vi "Trauma Box Controller.vi"() -> ()   [LabVIEW 2020]
uses:
  epl-vi-lib/Utility VIs/Buttons/KCheckmarkBoolean.ctl
  epl-vi-lib/Utility VIs/Controls/KBackground Gradient/KBackground Gradient.xctl
  Typedefs/TB-Parameters.ctl
  Typedefs/TB-Slack State.ctl
  epl-vi-lib/PXI DAQ VIs/AIDI/Typedefs/AIDI-Action.ctl
  epl-vi-lib/PXI DAQ VIs/AODO/Typedefs/AODO-Action.ctl
  Typedefs/TB-State Enum.ctl
  <vilib>/Analysis/baseanly.llb/Mean (DBL).vi
  <vilib>/Analysis/5stat.llb/RMS (DBL).vi
  epl-vi-lib/Utility VIs/Math VIs/Linear to dB (scalar).vi
  <vilib>/Analysis/NI_AALPro.lvlib
  <vilib>/Analysis/NI_AALBase.lvlib
panel:
  out "Exposure":errorcluster
  out "Crown":errorcluster
  in  "Waveform":u16(ring)=2 items=["Noise", "File", "Tone"]
  in  "dB SPL":dbl=100.0
  in  "Duration (min)":dbl=120.0
  in  "Tab Control":enum32{"Tone", "Noise", "File"}(tab)
  in  "Frequency (kHz)":dbl=8.0
  in  "High cutoff (kHz)":dbl=16.0
  in  "Low cutoff (kHz)":dbl=8.0
  in  "refWAV":path caption="Ref"
  in  "WAVfile":path
  in  "Cal Log":path=path "C:/Data/Trauma Box/Trauma Box Calibration Log.txt"
  out "Pistonphone Factor":dbl=102.0 caption="Calibrator Voltage\n(dB rms re 1 uV)"
  in  "B&K Mic Gain":dbl=20.0
  in  "Display":enum32{"Page 1", "Page 2"}(tab)
  out "ma":dbl=99.37258874088361 caption="average" format="%.1f"
  out "Starts":i32
  out "Overload 2":bool caption="Overload"
  in  "Fine Control":dbl(slide) caption="Fine Adjust (dB)" scale=-6.0..6.0
  out "Spectrum":waveform(dbl)(graph)
  out "Waveform":waveform(dbl)(graph)
  out "dB SPL rms":dbl=99.37258874088361 format="%.2f"
  out "Gauge":dbl(knob)=99.37258874088361 scale=80.0..130.0
  out "Elapsed time":string
  out "SPL History":cluster{dbl[], dbl[]}[](graph)
  out "Expected":string="Expected value = 102"
  in  "micCorrFile":path
  in  "Use mic correction":T1 caption="Apply mic frequency correction (if you're unsure, then no)"
  out "Calibration Log":string[][](table)
  out "Overload":bool
  out "Calibrator Voltage\n(dB rms re 1 uV)":dbl=-inf
  out "Pistonphone\nWaveform":dbl[](graph)
  in  "Wizard":T2(tab)
  in  "START":bool
  in  "EXIT":bool
  in  "Use previous":bool
  in  "Remeasure":bool
  in  "Pistonphone measure":bool
  in  "Next":bool
  in  "To Crown adjust":bool
  in  "Start Crown":bool
  in  "Stop Crown":bool
  in  "Start Trauma":bool
  in  "Stop Trauma":bool
  in  "Finished":bool
  in  "User ID":string
  in  "Gradient":dbl(xcontrol)
  # "dB SPL"
  # "Press START to begin\nPress EXIT to quit"
  # "Step 1 Pistonphone correction"
  # "Step 1 Pistonphone correction\n    \n--Put ref mic into pistonphone\n--Make sure B&K gain is correct"
  # "Step 2 Put microphone in cage. It's going to get loud! Close the booth door before continuing."
  # "Step 3 Adjust amplifier until SPL is correct, then hit \"Stop\" button:"
  # "Step 4: Noise Exposure\n1. Put animal(s) in cage\n2. Set duration,\n3. Press START"
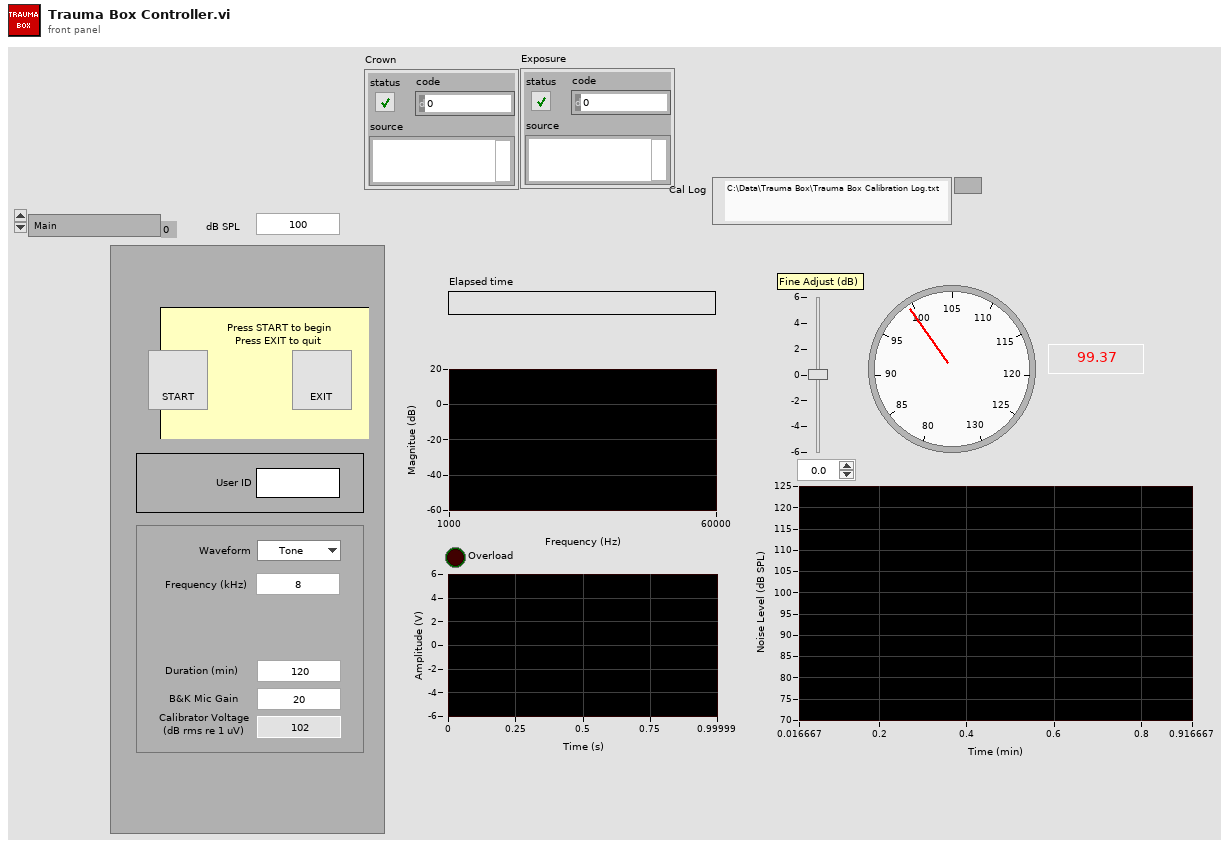
[diagram p1: front panel]
types:
  T1 = typedef "KCheckmarkBoolean.ctl" = bool
  T2 = enum32{"Main", "Pistonphone query", "Pistonphone measure", "Mic in cage", "Adjust Crown", "Animal in cage"}
  T3 = typedef "TB-Slack State.ctl" = cluster{"access_token":string, "bot id":string, "users":cluster{"id":string, "always":bool}[], "chan id":string}
  T4 = typedef "TB-Parameters.ctl" = cluster{"Low cutoff (kHz)":dbl, "High cutoff (kHz)":dbl, "Duration (min)":dbl, "dB SPL":dbl, "Waveform":enum16{"Noise", "File", "Tone"}, "WAVfile":path, "refWav":path, "use mic correction":bool, "micCorrFile":path, "Pistonphone Level (dB SPL)":dbl, "Sampling rate (Hz)":dbl, "Buffer length (s)":dbl, "Stream mic":bool, "Fine adjust":cluster{"Max":dbl, "Min":dbl}, "Mic gain":dbl, "atten":dbl, "resol (Hz)":dbl, "navgs":i32, "Allow Slack":bool, "max starts":i32, "Freq (kHz)":dbl, "Tma (s)":dbl, "Streamed":cluster{"Device":string, "Name":string}[], "Drive":string, "Speaker":string, "Mic":string}
  T5 = cluster{bool, "Exposure parameters":T4, "Slack":T3}
  T6 = typedef "AIDI-Action.ctl" = enum16{"Configure", "Initialize", "Start", "Read", "Clean up", "Init & Start", "Config & Test", "Position"}
  T7 = typedef "AODO-Action.ctl" = enum16{"Configure", "Initialize", "Start", "Write", "Clean up", "Init & Start", "Config & Test", "Position", "Set AO Gains", "Zero"}
  T8 = typedef "TB-Runtime state.ctl" = cluster{"stimfile":T9, "stream mic?":bool, "Fs":dbl, "ID":string, "micCorr":dbl[], "navg":i32, "r2sum":dbl[], "expose":bool, "spectra/frame":i32, "pts/spectra":i32, "nacq":i32, "init error":bool, "max starts":i32, "num starts":i32, "Setup":T10, "toneIndex":i32, "LastN":dbl[], "fine":dbl, "imic":i32, "stream":refnum<file>, "names":string[]}
  T9 = typedef "Sound File Refnum.ctl" = refnum<file>
  T10 = typedef "TB-Setup Log.ctl" = cluster{"Pistonphone factor":dbl, "Fine adjust":dbl, "Actual dB SPL":dbl, "Freq":dbl[], "Mag":dbl[]}
  T11 = typedef "TB-Stimulus State.ctl" = cluster{"filelen":i32, "stimfile":T9, "stimfile?":bool, "Fs":dbl, "Npts":i32, "stimfileend":bool, "atten":dbl, "AO":i32[]}
  T12 = typedef "TB-Log.ctl" = cluster{"Slack":T3, "entries":string[]}
  T13 = typedef "TB-Mic Queue.ctl" = refnum<queue>
  T14 = typedef "TB-State Enum.ctl" = enum16{"Main", "Pistonphone query", "Pistonphone measure", "Mic in cage", "Adjust Crown", "Animal in cage"}
  T15 = cluster{"notification":bool, "Parameters out":T4, "Slack":T3}
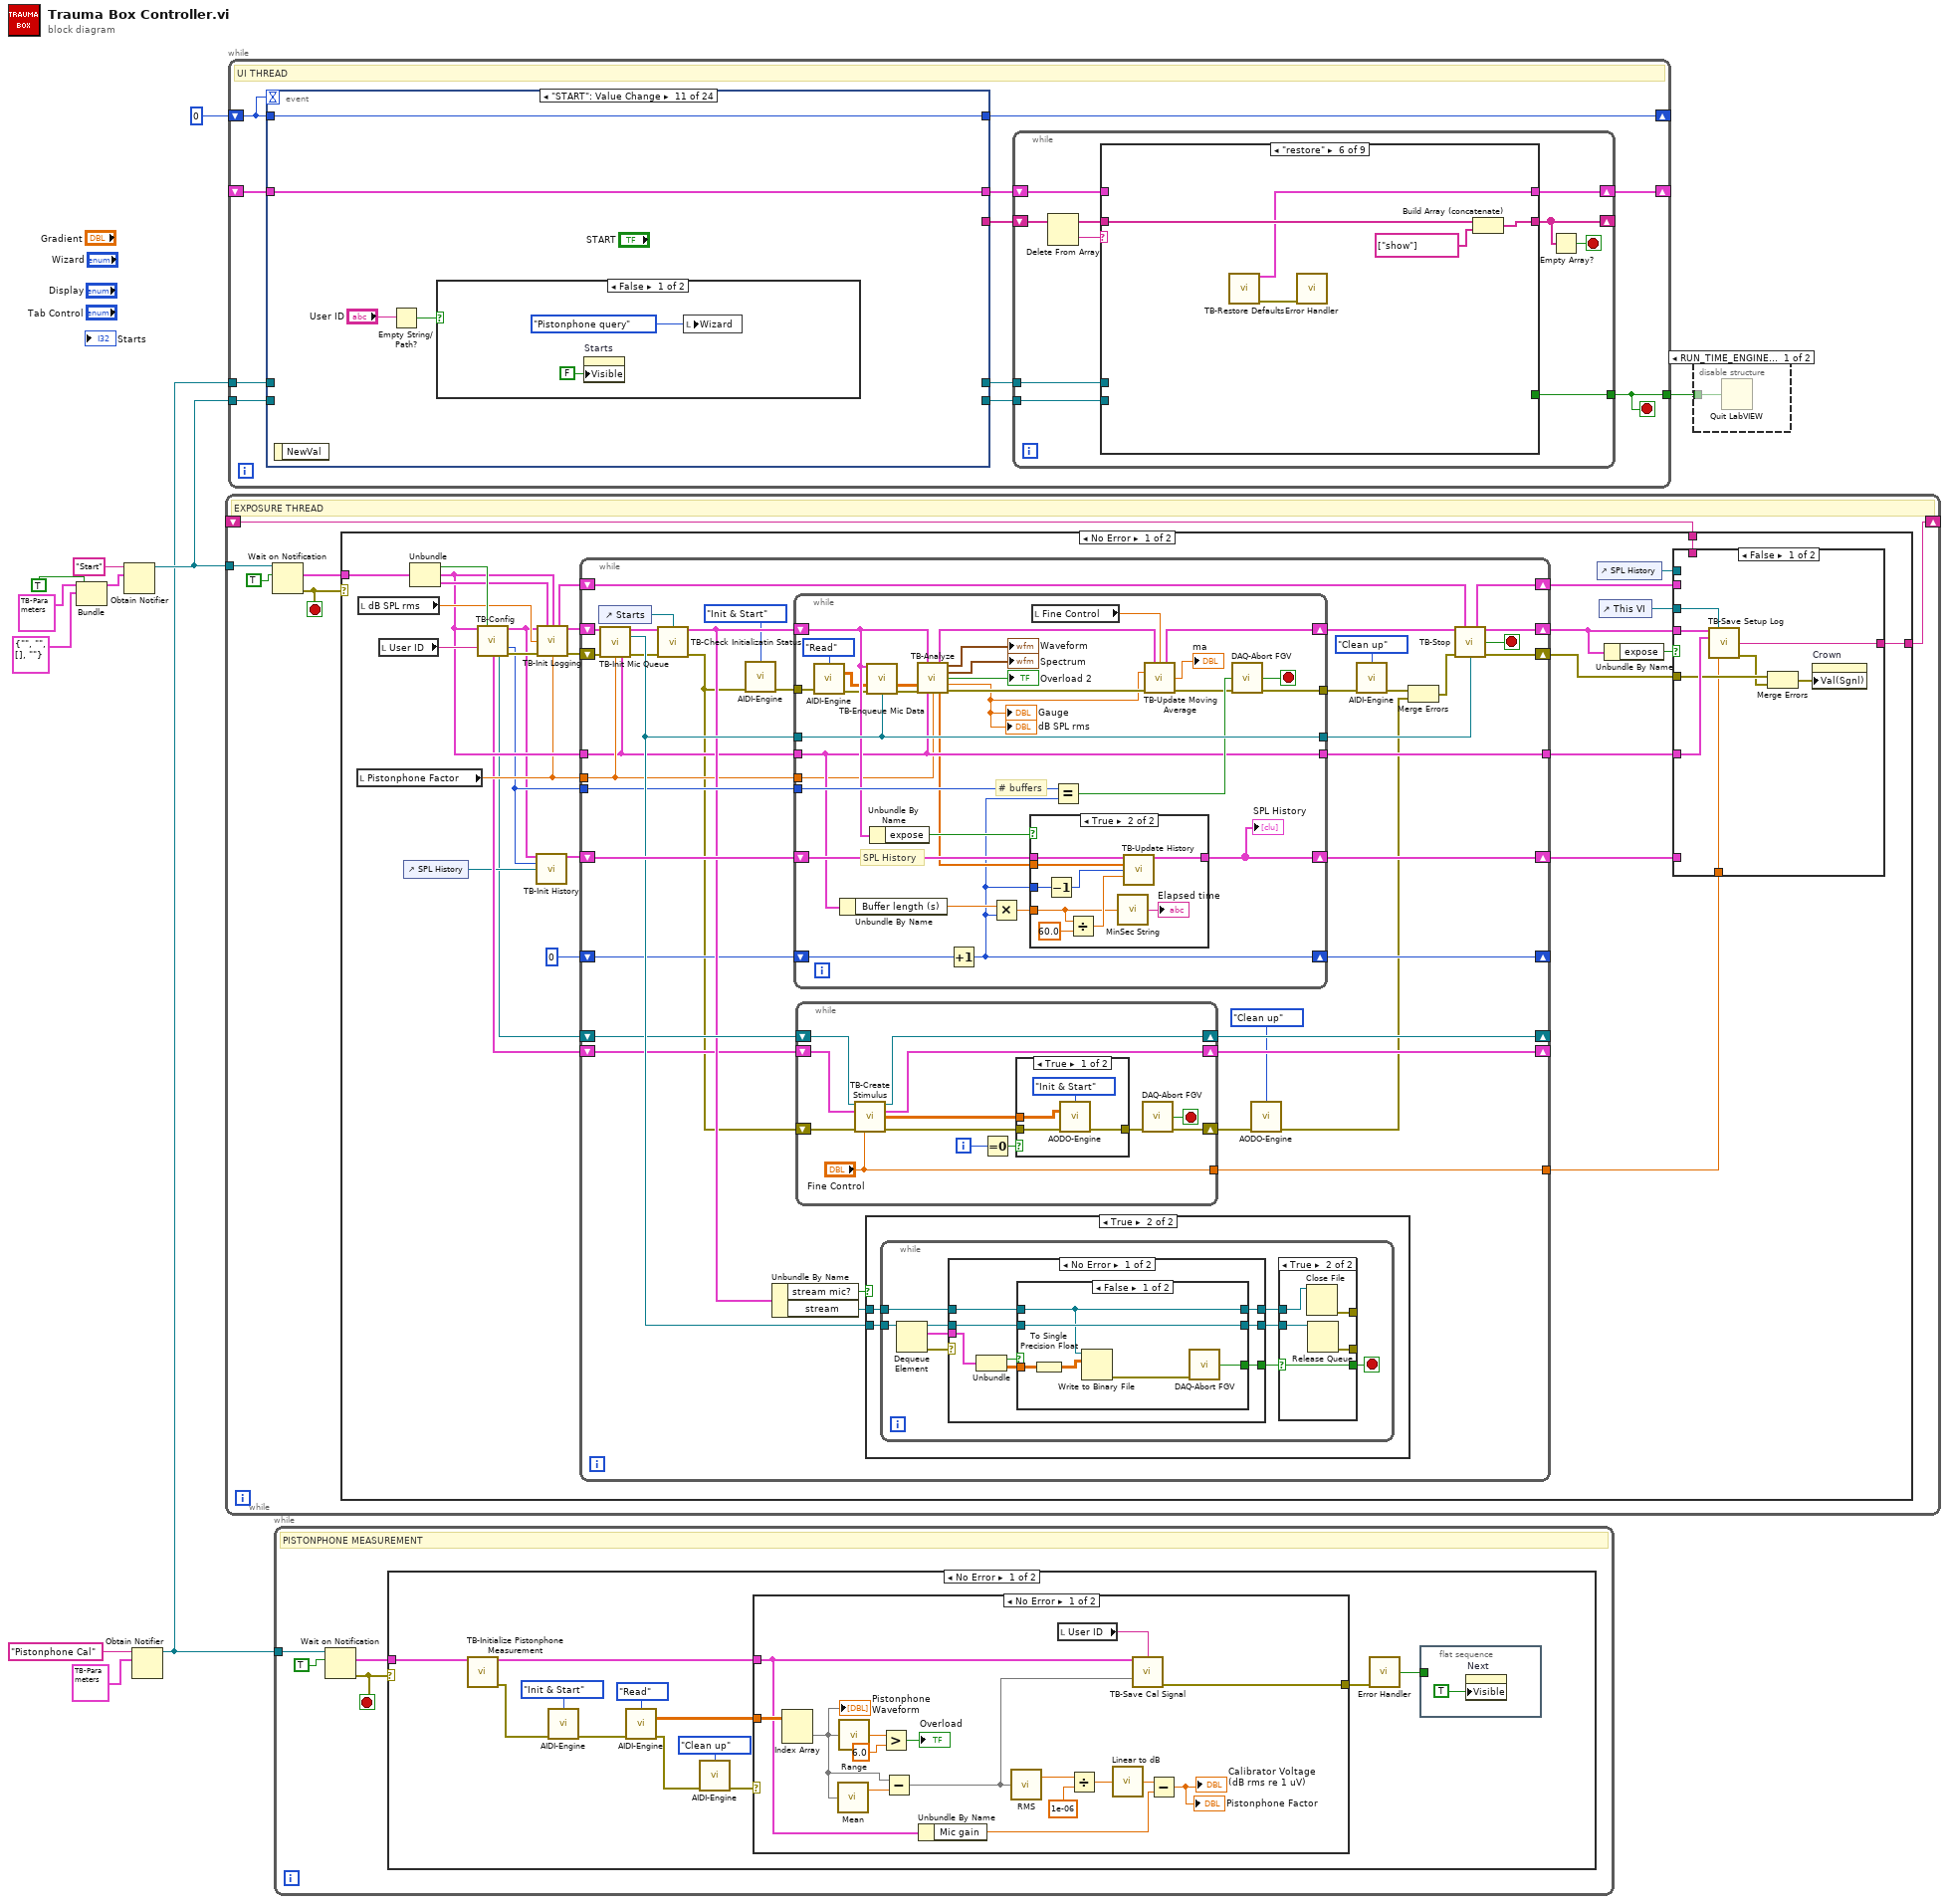
[diagram p0: block diagram]
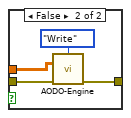
[diagram p3: hidden frame]
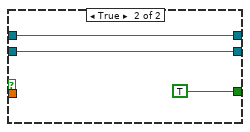
[diagram p6: hidden frame]
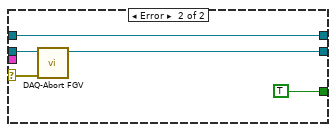
[diagram p7: hidden frame]
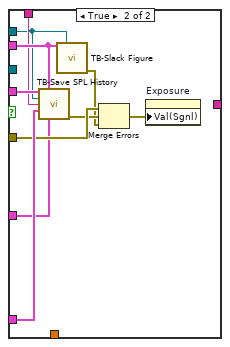
[diagram p8: hidden frame]
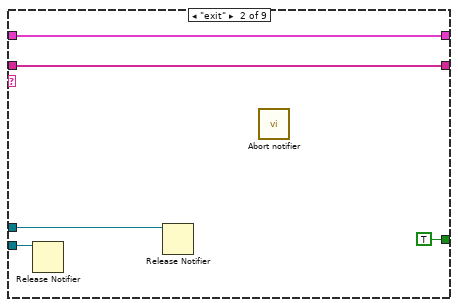
[diagram p11: hidden frame]
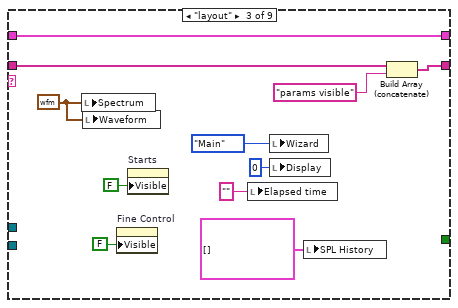
[diagram p12: hidden frame]
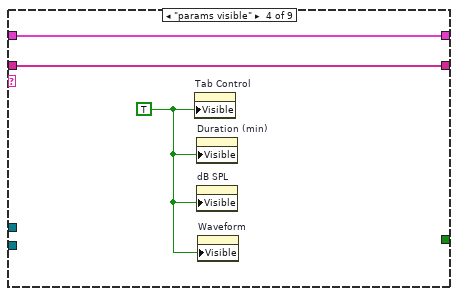
[diagram p13: hidden frame]
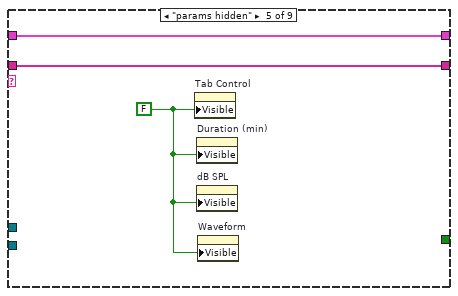
[diagram p14: hidden frame]
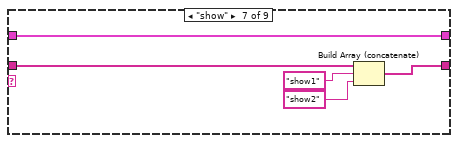
[diagram p15: hidden frame]
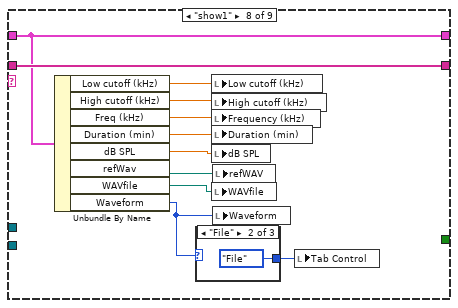
[diagram p16: hidden frame]
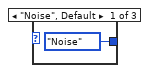
[diagram p17: hidden frame]
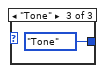
[diagram p18: hidden frame]
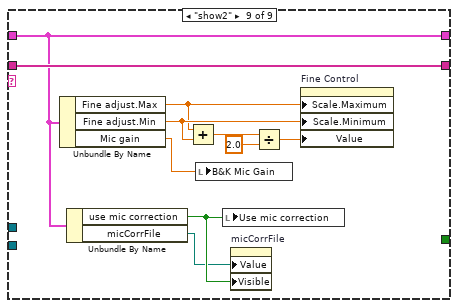
[diagram p19: hidden frame]
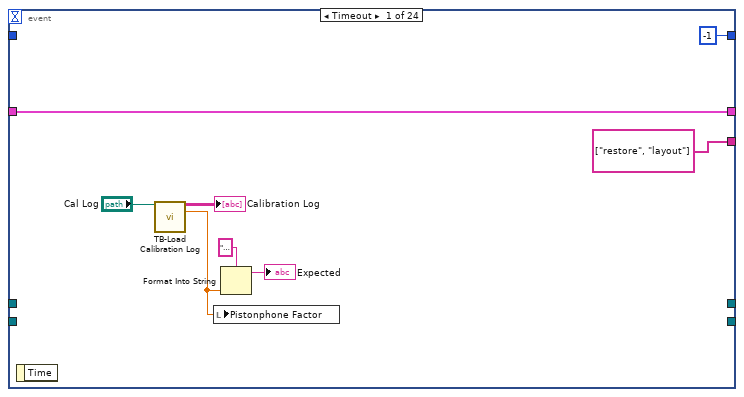
[diagram p20: hidden frame]
diagram:
  n1 = Bundle(TRUE, "Exposure parameters"=T4 {"Low cutoff (kHz)"=0.0, "High cutoff (kHz)"=0.0, "Duration (min)"=0.0, "dB SPL"=0.0, "Waveform"=enum."Noise", "WAVfile"=path "", "refWav"=path "", "use mic correction"=FALSE, "micCorrFile"=path "", "Pistonphone Level (dB SPL)"=0.0, "Sampling rate (Hz)"=0.0, "Buffer length (s)"=0.0, "Stream mic"=FALSE, "Fine adjust"={"Max"=0.0, "Min"=0.0}, "Mic gain"=0.0, "atten"=0.0, "resol (Hz)"=0.0, "navgs"=0, "Allow Slack"=FALSE, "max starts"=0, "Freq (kHz)"=8.0, "Tma (s)"=0.0, "Streamed"=[], "Drive"="", "Speaker"="", "Mic"=""}, "Slack"=T3 {"access_token"="", "bot id"="", "users"=[], "chan id"=""}) -> (w3:T5)  [unwired: 1 in]
  n2 = Obtain Notifier(name (unnamed)="Start", notification data type=w3) -> (notifier out=w11:refnum<notifier>)  [unwired: 2 in, 2 out]
  n3 = Obtain Notifier(name (unnamed)="Pistonphone Cal", notification data type=T4 {"Low cutoff (kHz)"=114.0, "High cutoff (kHz)"=100000.0, "Duration (min)"=1.0, "dB SPL"=100.0, "Waveform"=enum."Noise", "WAVfile"=path "", "refWav"=path "", "use mic correction"=FALSE, "micCorrFile"=path "", "Pistonphone Level (dB SPL)"=0.0, "Sampling rate (Hz)"=0.0, "Buffer length (s)"=0.0, "Stream mic"=FALSE, "Fine adjust"={"Max"=0.0, "Min"=0.0}, "Mic gain"=0.0, "atten"=0.0, "resol (Hz)"=0.0, "navgs"=0, "Allow Slack"=FALSE, "max starts"=0, "Freq (kHz)"=8.0, "Tma (s)"=0.0, "Streamed"=[], "Drive"="", "Speaker"="", "Mic"=""} ("Exposure parameters")) -> (notifier out=w7:refnum<notifier>)  [unwired: 2 in, 2 out]
  n4 = while {
    tunnel: w11 -> [w16]
    shift-right: [w13] -> _
    shift-left: _ -> [w12]
    stop <- w15 stop-if-true
    # "EXPOSURE THREAD"
    n5 = Wait on Notification(notifier=w16, ignore previous (F)=TRUE) -> (notification=w14:T5, error out=w15:errorcluster)  [unwired: 2 in, 2 out]
    n6 = case shown="No Error" w15 {
      tunnel: w14 -> [w46 _]
      tunnel: [w25 _] -> w13
      tunnel: w12 -> [w24 _]
      frame No Error {
        n7 = local read "Pistonphone Factor"() -> (w28:dbl)
        n8 = local read "dB SPL rms"() -> (w36:dbl)
        n9 = local read "User ID"() -> (w44:string)
        n10 = control-ref of="SPL History"() -> (w22:refnum<vi>)
        n11 = Unbundle(w46) -> (w45:bool, "Exposure parameters"=w35:T4, "Slack"=w38:T3)
        n12 = call "TB-Config.vi"("Params"=w35, "Exposure?"=w45, "ID"=w44) -> ("state"=w20:T8, "Num Buffers"=w21:i32, "stimulus state"=w23:T11, "SigMan"=w18:refnum<class "SignalManager.lvclass">, "error out"=w40:errorcluster)  [unwired: 8 in]
        n13 = call "TB-Init History.vi"("state"=w20, "Num Buffers"=w21, "XYGraph in"=w22) -> ("history"=w19:cluster{dbl[], dbl[]}[])  [unwired: 12 in]
        n14 = call "TB-Init Logging.vi"("state in"=w20, "Slack"=w38, "Params"=w35, "Level"=w36, "error in (no error)"=w40, "Pistonphone factor"=w28) -> ("Log"=w33:T12, "state out"=w37:T8, "error out"=w39:errorcluster)  [unwired: 7 in]
        n15 = while {
          tunnel: w28 -> [w58]
          tunnel: w21 -> [w79]
          tunnel: w35 -> [w57]
          shift-right: [w81] -> w43
          shift-left: w19 -> [w85]
          shift-right: [w76] -> w41
          shift-left: w39 -> [w75]
          shift-right: [w73] -> w34
          shift-left: w37 -> [w74]
          shift-right: [w71] -> w32
          shift-left: w33 -> [w72]
          shift-right: [w65] -> _
          shift-left: 0 -> [w66]
          shift-right: [w64] -> _
          shift-left: w18 -> [w80]
          shift-right: [w62] -> _
          shift-left: w23 -> [w61]
          tunnel: [w60] -> w29
          tunnel: [w59] -> w27
          stop <- w67 stop-if-true
          n16 = control-ref of="Starts"() -> (w63:refnum<vi>)
          n17 = call "TB-Init Mic Queue.vi"("state in"=w74, "error in (no error)"=w75, "Pistonphone factor"=w58, "Exposure parameters"=w57) -> ("state out"=w69:T8, "mic queue"=w84:T13, "error out"=w70:errorcluster)  [unwired: 9 in]
          n18 = call "TB-Check Initializatin Status.vi"("state in"=w69, "Starts"=w63, "error in (no error)"=w70) -> ("state out"=w68:T8, "error out"=w47:errorcluster)  [unwired: 11 in]
          n19 = call "AIDI-Engine.vi"("Action"=AIDI-Action."Init & Start", "error in (no error)"=w47) -> ("error out"=w49:errorcluster)  [unwired: 10 in, 3 out]
          n20 = Unbundle By Name(w68) -> ("stream mic?"=w78:bool, "stream"=w83:refnum<file>)
          n21 = while {
            tunnel: w79 -> [w117]
            shift-right: [w112] -> w81
            shift-left: w85 -> [w114]
            tunnel: w58 -> [w92]
            tunnel: w57 -> [w100]
            tunnel: w84 -> [w107]
            tunnel: [w107] -> w82
            shift-right: [w96] -> w77
            shift-left: w68 -> [w104]
            tunnel: [w105] -> w51
            shift-right: [w90] -> w65
            shift-left: w66 -> [w101]
            tunnel: [w100] -> w60
            tunnel: w49 -> [w86]
            stop <- w106 stop-if-true
            # "# buffers"
            # "SPL History"
            n22 = call "AIDI-Engine.vi"("Action"=AIDI-Action."Read", "error in (no error)"=w86) -> ("AI"=w88:dbl[][], "error out"=w89:errorcluster)  [unwired: 10 in, 2 out]
            n23 = Unbundle By Name(w100) -> ("Buffer length (s)"=w110:dbl)
            n24 = call "TB-Enqueue Mic Data.vi"("state thru"=w104, "AI Waveforms in"=w88, "error in (no error)"=w89, "Queue in"=w107) -> ("AI Waveforms thru"=w109:dbl[][], "error out"=w108:errorcluster)  [unwired: 10 in]
            n25 = Unbundle By Name(w104) -> ("expose"=w103:bool)
            n26 = call "TB-Analyze.vi"("state in"=w104, "AI Waveforms"=w109, "error in (no error)"=w108, "Exposure parameters"=w100, "Pistonphone Factor"=w92) -> ("state out"=w97:T8, "waveform"=→"Waveform":waveform(dbl), "spectrum"=→"Spectrum":waveform(dbl), "Overload"=→"Overload 2":bool, "Cal SPL"=w94:dbl, "history values"=w91:dbl[], "error out"=w99:errorcluster)  [unwired: 4 in]
            "Gauge" <- w94
            "dB SPL rms" <- w94
            n27 = Increment(x=w101) -> (x+1=w90:i32)
            n28 = Multiply(x=w110, y=w90) -> (x*y=w115:dbl)
            n29 = case shown="True" w103 {
              tunnel: w115 -> [_ w119]
              tunnel: w114 -> [w118 w125]
              tunnel: [w118 w124] -> w112
              tunnel: w91 -> [_ w123]
              tunnel: w90 -> [_ w122]
              frame False {
              }
              frame True {
                n30 = Decrement(x=w122) -> (x-1=w121:i32)
                n31 = Divide(x=w119, y=60.0) -> (x/y=w120:dbl)
                n32 = call "MinSec String.vi"("Seconds"=w119) -> ("MinSec string"=→"Elapsed time":string)
                n33 = call "TB-Update History.vi"("history in"=w125, "history values"=w123, "Index"=w121, "Time"=w120) -> ("history out"=w124:cluster{dbl[], dbl[]}[])  [unwired: 11 in]
              }
            }
            "SPL History" <- w112
            n34 = local read "Fine Control"() -> (w93:dbl)
            n35 = Equal?(x=w117, y=w90) -> (x = y?=w102:bool)
            n36 = call "TB-Update Moving Average.vi"("state in"=w97, "fine"=w93, "SPL"=w94, "error in (no error)"=w99) -> ("state out"=w96:T8, "moving average"=→"ma":dbl, "error out"=w98:errorcluster)  [unwired: 9 in]
            n37 = call "DAQ-Abort FGV.vi"("Finished"=w102, "error in (no error)"=w98) -> ("Stop"=w106:bool, "Errors"=w105:errorcluster)  [unwired: 11 in, 1 out]
          }
          n38 = while {
            shift-right: [w129] -> w55
            shift-left: w47 -> [w138]
            shift-right: [w137] -> w64
            shift-left: w80 -> [w139]
            shift-right: [w134] -> w62
            shift-left: w61 -> [w140]
            tunnel: ["Fine Control"] -> w59
            i -> [w135]
            stop <- w128 stop-if-true
            n39 = call "TB-Create Stimulus.vi"("StimChan In"=w139, "state"=w140, "error in (no error)"=w138, "Fine adjust (dB)"="Fine Control") -> ("StimChan Out"=w137:refnum<class "SignalManager.lvclass">, "state out"=w134:T11, "Stimulus"=w132:dbl[][], "error out"=w131:errorcluster)  [unwired: 8 in]
            n40 = Equal To 0?(x=w135) -> (x = 0?=w136:bool)
            n41 = case shown="True" w136 {
              tunnel: w131 -> [w144 w148]
              tunnel: [w143 w147] -> w130
              tunnel: w132 -> [w141 w145]
              frame True {
                n42 = call "AODO-Engine.vi"("Action"=AODO-Action."Init & Start", "AO"=w141, "error in (no error)"=w144) -> ("error out"=w143:errorcluster)  [unwired: 11 in, 1 out]
              }
              frame False {
                n43 = call "AODO-Engine.vi"("Action"=AODO-Action."Write", "AO"=w145, "error in (no error)"=w148) -> ("error out"=w147:errorcluster)  [unwired: 11 in, 1 out]
              }
            }
            n44 = call "DAQ-Abort FGV.vi"("error in (no error)"=w130) -> ("Stop"=w128:bool, "Errors"=w129:errorcluster)  [unwired: 12 in, 1 out]
          }
          n45 = case shown="True" w78 {
            tunnel: w84 -> [_ w150]
            tunnel: w83 -> [_ w149]
            frame False {
            }
            frame True {
              n46 = while {
                tunnel: w150 -> [w159]
                tunnel: w149 -> [w153]
                stop <- w154 stop-if-true
                n47 = Dequeue Element(queue=w159) -> (queue out=w156:T13, element=w157:cluster{bool, dbl[][]}, error out=w158:errorcluster)  [unwired: 2 in, 1 out]
                n48 = case shown="No Error" w158 {
                  selector: w158 -> [_ w183]
                  tunnel: w157 -> [w173 _]
                  tunnel: [w171 TRUE ("status")] -> w155
                  tunnel: w156 -> [w169 w184]
                  tunnel: w153 -> [w168 w185]
                  tunnel: [w167 w185] -> w152
                  tunnel: [w166 w184] -> w151
                  frame No Error {
                    n49 = Unbundle(w173) -> (w172:bool, w170:dbl[][])
                    n50 = case shown="False" w172 {
                      tunnel: [w178 TRUE ("status")] -> w171
                      tunnel: w170 -> [w175 _]
                      tunnel: w169 -> [w179 w180]
                      tunnel: w168 -> [w177 w181]
                      tunnel: [w177 w181] -> w167
                      tunnel: [w179 w180] -> w166
                      frame False {
                        n51 = To Single Precision Float(number=w175) -> (single precision float=w174:sgl[][])
                        n52 = Write to Binary File(file (use dialog)=w177, data=w174) -> (error out=w176:errorcluster)  [unwired: 4 in, 2 out]
                        n53 = call "DAQ-Abort FGV.vi"("error in (no error)"=w176) -> ("Stop"=w178:bool)  [unwired: 12 in, 2 out]
                      }
                      frame True {
                      }
                    }
                  }
                  frame Error {
                    n54 = call "DAQ-Abort FGV.vi"("error in (no error)"=w183) -> ()  [unwired: 12 in, 3 out]
                  }
                }
                n55 = case shown="True" w155 {
                  selector: w155 -> [w160 w165]
                  tunnel: [w160 w165] -> w154
                  tunnel: w152 -> [_ w162]
                  tunnel: w151 -> [_ w164]
                  tunnel: [_ w163] -> _
                  tunnel: [_ w161] -> _
                  frame False {
                  }
                  frame True {
                    n56 = Close File(refnum=w162) -> (error out=w161:errorcluster)  [unwired: 1 in, 1 out]
                    n57 = Release Queue(queue=w164) -> (error out=w163:errorcluster)  [unwired: 2 in, 2 out]
                  }
                }
              }
            }
          }
          n58 = call "AODO-Engine.vi"("Action"=AODO-Action."Clean up", "error in (no error)"=w55) -> ("error out"=w53:errorcluster)  [unwired: 12 in, 1 out]
          n59 = call "AIDI-Engine.vi"("Action"=AIDI-Action."Clean up", "error in (no error)"=w51) -> ("error out"=w52:errorcluster)  [unwired: 10 in, 3 out]
          n60 = Merge Errors(w52, w53) -> (w50:errorcluster)
          n61 = call "TB-Stop.vi"("state in"=w77, "Log in"=w72, "error in (no error)"=w50, "Queue in"=w82) -> ("Log out"=w71:T12, "state out"=w73:T8, "Finished"=w67:bool, "error out"=w76:errorcluster)  [unwired: 8 in]
        }
        n62 = control-ref of="SPL History"() -> (w30:refnum<vi>)
        n63 = control-ref of="This VI"() -> (w26:refnum<vi>)
        n64 = Unbundle By Name(w34) -> ("expose"=w42:bool)
        n65 = case shown="False" w42 {
          tunnel: w43 -> [_ w204]
          tunnel: w34 -> [w193 w203]
          tunnel: w41 -> [w192 w202]
          tunnel: w32 -> [_ w198]
          tunnel: w30 -> [_ w196]
          tunnel: w29 -> [w194 w195]
          tunnel: w27 -> [w189 _]
          tunnel: w26 -> [w188 _]
          tunnel: [w187 _] -> w25
          tunnel: w24 -> [_ w197]
          frame False {
            n66 = call "TB-Save Setup Log.vi"("State"=w193, "VI ref"=w188, "Exposure parameters"=w194, "Fine Control"=w189) -> ("date/time string"=w187:string, "error out"=w190:errorcluster)  [unwired: 10 in]
            n67 = Merge Errors(w192, w190) -> (w191:errorcluster)
            n68 = property on="Crown" class="Clust (strict)"("Val(Sgnl)"=w191) -> ()  [unwired: 2 in, 2 out]
          }
          frame True {
            n69 = call "TB-Save SPL History.vi"("state"=w203, "Log in"=w198, "XYGraph in"=w196, "date/time string"=w197, "history"=w204, "Exposure parameters"=w195) -> ("error out"=w200:errorcluster)  [unwired: 9 in]
            n70 = call "TB-Slack Figure.vi"("Log"=w198, "XYGraph in"=w196) -> ("error out"=w199:errorcluster)  [unwired: 13 in]
            n71 = Merge Errors(w202, w200, w199) -> (w201:errorcluster)
            n72 = property on="Exposure" class="Clust (strict)"("Val(Sgnl)"=w201) -> ()  [unwired: 2 in, 2 out]
          }
        }
      }
      frame Error {
      }
    }
  }
  n73 = while {
    tunnel: w11 -> [w215]
    shift-right: [w214] -> _
    shift-left: 0 -> [w211]
    tunnel: w7 -> [w213]
    tunnel: [w205] -> w6
    shift-right: [w206] -> _
    shift-left: _ -> [w212]
    stop <- w205 stop-if-true
    # "UI THREAD"
    n74 = event shown="[10] \"START\": Value Change" {
      selector: _ -> [_ _ _ _ _ _ _ _ _ _ _ _ _ _ _ _ _ _ _ _ _ _ _ _]
      dyn-events: _ -> [_ _ _ _ _ _ _ _ _ _ _ _ _ _ _ _ _ _ _ _ _ _ _ _]
      timeout: w211 -> [_ _ _ _ _ _ _ _ _ _ _ _ _ _ _ _ _ _ _ _ _ _ _ _]
      tunnel: w215 -> [_ w292 w299 _ _ _ _ _ _ _ _ _ _ _ _ w398 w406 _ w441 _ _ w462 _ _]
      tunnel: [_ w292 w299 _ _ _ _ _ _ _ _ _ _ _ _ _ _ _ _ _ _ w462 _ _] -> w208
      tunnel: [-1 w295 w303 w328 w334 w340 w343 w348 w356 w357 w362 w369 w373 w379 w382 w391 w402 w414 w424 w453 w455 w459 w466 w470] -> w214
      tunnel: w213 -> [_ w293 w300 _ _ _ _ _ _ _ _ _ _ w380 _ _ _ _ _ _ _ w461 _ _]
      tunnel: [_ w293 w300 _ _ _ _ _ _ _ _ _ _ _ _ _ _ _ _ _ _ w461 _ _] -> w209
      tunnel: [w288 w296 w301 w329 w337 w341 w346 w351 w354 w360 w363 w370 w374 w378 w383 w388 w403 w415 w422 w454 w456 w460 w465 w469] -> w207
      tunnel: w212 -> [w288 w296 w304 w330 w338 w342 w347 w352 w355 w361 w363 w370 w374 w378 w383 w388 w403 w415 w422 w454 w456 w460 w465 w469]
      tunnel: w211 -> [_ w295 w303 w328 w334 w340 w343 w348 w356 w357 w362 w369 w373 w379 w382 w391 w402 w414 w424 w453 w455 w459 w466 w470]
      tunnel: [string[] ["restore", "layout"] string[] ["exit"] w302 _ _ _ _ _ _ _ _ _ string[] ["params hidden"] _ string[] ["params visible"] _ _ _ _ _ _ string[] ["exit"] _ _] -> w210
      event Timeout {
        n75 = event-data() -> ()  [unwired: 1 in, 1 out]
        n76 = call "TB-Load Calibration Log.vi"("Cal Log"="Cal Log") -> ("Log"=→"Calibration Log":string[][], "mean value"=w286:dbl)  [unwired: 13 in]
        n77 = local write "Pistonphone Factor"(w286) -> ()
        n78 = Format Into String(format string="Expected value = %d", w286) -> (resulting string=→"Expected":string)  [unwired: 2 in, 1 out]
      }
      event Panel Close? {
        n79 = event-data() -> ()  [unwired: 1 in, 1 out]
        n80 = event-data("Discard?"=TRUE) -> ()  [unwired: 1 in, 1 out]
      }
      event Menu Selection (User) {
        n81 = event-data() -> ("ItemTag"=w305:string)  [unwired: 1 in]
        n82 = case shown="\"mmEditOptions\"" w305 {
          tunnel: [_ _ w314 _ _ _] -> w298
          tunnel: w304 -> [w306 w307 w311 w320 w322 w324]
          tunnel: [w306 w307 w310 w320 w322 w325] -> w301
          tunnel: [_ string[] ["restore"] _ string[] ["restore", "layout"] string[] ["exit"] _] -> w302
          frame "", Default {
          }
          frame "mmFileRestore" {
          }
          frame "mmFileSave" {
            n83 = property on="Fine Control" class="Slide (strict)"() -> ("Scale.Maximum"=w313:dbl, "Scale.Minimum"=w312:dbl)  [unwired: 2 in, 2 out]
            n84 = Bundle By Name(cluster=w311, "Fine adjust.Max"=w313, "Fine adjust.Min"=w312) -> (w310:T4)
            n85 = call "Default Config File Path.vi"() -> ("Default config file name"=w316:path)
            n86 = call "Write Anything.vi"("Section Name (Name of \"Anything\")"="Params" ("Section Name (Name of \"Anything\")"), "Anything"=w310, "Path (dialog)"=w316) -> ("Error Out"=w315:errorcluster)  [unwired: 7 in, 1 out]
            n87 = case shown="No Error" w315 {
              selector: w315 -> [_ w318]
              tunnel: [_ w318] -> w314
              frame No Error {
                n88 = One Button Dialog(message="Defaults saved.") -> ()  [unwired: 1 in, 1 out]
              }
              frame Error {
              }
            }
          }
          frame "mmFileRestart" {
          }
          frame "mmFileExit" {
          }
          frame "mmEditOptions" {
            n89 = control-ref of="This VI"() -> (w323:refnum<vi>)
            n90 = call "TB-Options Dialog.vi"("Parameters in"=w324, "Parent VI"=w323) -> ("Parameters out"=w325:T4)  [unwired: 12 in, 1 out]
          }
        }
        n91 = call "Error Handler.vi"("error in (no error)"=w298) -> ()  [unwired: 13 in, 2 out]
      }
      event "Waveform": Value Change {
        n92 = event-data() -> ()  [unwired: 1 in, 1 out]
        n93 = case shown="1" "Waveform" {
          tunnel: [enum32{"Tone", "Noise", "File"}."Noise" ("Tab Control") enum32{"Tone", "Noise", "File"}."File" ("Tab Control") enum32{"Tone", "Noise", "File"}."Tone" ("Tab Control")] -> w327
          frame 2, Default {
          }
          frame 4 {
          }
          frame 1 {
          }
        }
        n94 = local write "Tab Control"(w327) -> ()
        n95 = Bundle By Name(cluster=w330, "Waveform"="Waveform") -> (w329:T4)
      }
      event "Low cutoff (kHz)", "High cutoff (kHz)": Value Change {
        n96 = event-data() -> ()  [unwired: 1 in, 1 out]
        n97 = Bundle By Name(cluster=w338, "Low cutoff (kHz)"="Low cutoff (kHz)", "High cutoff (kHz)"="High cutoff (kHz)") -> (w337:T4)
      }
      event "Frequency (kHz)": Value Change {
        n98 = event-data() -> ()  [unwired: 1 in, 1 out]
        n99 = Bundle By Name(cluster=w342, "Freq (kHz)"="Frequency (kHz)") -> (w341:T4)
      }
      event "WAVfile", "refWAV": Value Change {
        n100 = event-data() -> ()  [unwired: 1 in, 1 out]
        n101 = Bundle By Name(cluster=w347, "WAVfile"="WAVfile", "refWav"="refWAV") -> (w346:T4)
      }
      event "micCorrFile": Value Change {
        n102 = event-data() -> ()  [unwired: 1 in, 1 out]
        n103 = Bundle By Name(cluster=w352, "use mic correction"="Use mic correction", "micCorrFile"="micCorrFile") -> (w351:T4)
        n104 = property on="micCorrFile" class="Path"("Visible"="Use mic correction") -> ()  [unwired: 2 in, 2 out]
      }
      event "B&K Mic Gain": Value Change {
        n105 = event-data() -> ()  [unwired: 1 in, 1 out]
        n106 = Bundle By Name(cluster=w355, "Mic gain"="B&K Mic Gain") -> (w354:T4)
      }
      event "Duration (min)", "dB SPL": Value Change {
        n107 = event-data() -> ()  [unwired: 1 in, 1 out]
        n108 = Bundle By Name(cluster=w361, "Duration (min)"="Duration (min)", "dB SPL"="dB SPL") -> (w360:T4)
      }
      event "START": Value Change {
        n109 = event-data() -> ()  [unwired: 1 in, 1 out]
        n110 = Empty String/Path?(string/path="User ID") -> (empty?=w364:bool)
        n111 = case shown="False" w364 {
          frame False {
            n112 = property on="Starts" class="DigNum (strict)"("Visible"=FALSE) -> ()  [unwired: 2 in, 2 out]
            n113 = local write "Wizard"(TB-State_Enum."Pistonphone query" ("State")) -> ()
          }
          frame True {
            n114 = One Button Dialog(message="Please enter a User ID (for bookkeeping purposes).") -> ()  [unwired: 1 in, 1 out]
          }
        }
      }
      event "Use previous": Value Change {
        n115 = event-data() -> ()  [unwired: 1 in, 1 out]
        n116 = local write "Wizard"(TB-State_Enum."Mic in cage" ("State")) -> ()
      }
      event "Remeasure": Value Change {
        n117 = event-data() -> ()  [unwired: 1 in, 1 out]
        n118 = property on="Next" class="Bool"("Visible"=FALSE) -> ()  [unwired: 2 in, 2 out]
        n119 = local write "Display"(1) -> ()
        n120 = local write "Wizard"(TB-State_Enum."Pistonphone measure" ("State")) -> ()
      }
      event "Pistonphone measure": Value Change {
        n121 = event-data() -> ()  [unwired: 1 in, 1 out]
        n122 = Send Notification(notification=w378, notifier=w380) -> ()  [unwired: 1 in, 2 out]
      }
      event "Next": Value Change {
        n123 = event-data() -> ()  [unwired: 1 in, 1 out]
        n124 = local write "Wizard"(TB-State_Enum."Mic in cage" ("State")) -> ()
        n125 = local write "Display"(0) -> ()
      }
      event "To Crown adjust": Value Change {
        n126 = event-data() -> ()  [unwired: 1 in, 1 out]
        n127 = property on="Fine Control" class="Slide (strict)"("Visible"=TRUE, "Value"=0.0 ("Fine Control")) -> (error out=w393:errorcluster)  [unwired: 2 in, 1 out]
        n128 = local write "Elapsed time"("" ("Elapsed time")) -> ()
        n129 = local write "Wizard"(TB-State_Enum."Adjust Crown" ("State")) -> ()
        n130 = Bundle("notification"=FALSE, "Parameters out"=w388, "Slack"=T3 {"access_token"="", "bot id"="", "users"=[], "chan id"=""}) -> (w390:T15)  [unwired: 1 in]
        n131 = Send Notification(notification=w390, notifier=w398, error in (no error)=w393) -> ()  [unwired: 2 out]
        n132 = property on="Start Crown" class="Bool"("Visible"=FALSE) -> ()  [unwired: 2 in, 2 out]
        n133 = Unbundle By Name(w388) -> ("Tma (s)"=w387:dbl)
        n134 = Greater Than 0?(x=w387) -> (x > 0?=w386:bool)
        n135 = property on="ma" class="DigNum (strict)"("Visible"=w386) -> ()  [unwired: 2 in, 2 out]
      }
      event "Start Crown": Value Change {
        n136 = event-data() -> ()  [unwired: 1 in, 1 out]
        n137 = while {
          tunnel: w406 -> [w412]
          tunnel: [w408] -> w405
          stop <- w410 stop-if-true
          n138 = Get Notifier Status(notifier=w412) -> (notifier out=w408:refnum<notifier>, # waiting=w411:i32)  [unwired: 1 in, 3 out]
          n139 = Wait (ms)(milliseconds to wait=u32 250) -> ()  [unwired: 1 out]
          n140 = Greater Than 0?(x=w411) -> (x > 0?=w410:bool)
        }
        n141 = Bundle("notification"=FALSE, "Parameters out"=w403, "Slack"=T3 {"access_token"="", "bot id"="", "users"=[], "chan id"=""}) -> (w401:T15)  [unwired: 1 in]
        n142 = Send Notification(notification=w401, notifier=w405) -> ()  [unwired: 1 in, 2 out]
        n143 = property on="Start Crown" class="Bool"("Visible"=FALSE) -> ()  [unwired: 2 in, 2 out]
      }
      event "Stop Crown": Value Change {
        w416 = TRUE ("Visible")
        n144 = event-data() -> ()  [unwired: 1 in, 1 out]
        n145 = local write "Wizard"(TB-State_Enum."Animal in cage" ("State")) -> ()
        n146 = property on="Start Trauma" class="Bool"("Visible"=w416) -> ()  [unwired: 2 in, 2 out]
        n147 = property on="Stop Trauma" class="Bool"("Visible"=w416) -> ()  [unwired: 2 in, 2 out]
        n148 = call "DAQ-Abort FGV.vi"("Action"=enum16{"Default", "Init", "Abort", "1st error"}."Abort") -> ()  [unwired: 12 in, 3 out]
      }
      event "Start Trauma": Value Change {
        n149 = event-data() -> ("CtlRef"=w419:refnum<vi>)  [unwired: 1 in]
        n150 = local read "Pistonphone Factor"() -> (w435:dbl)
        n151 = Get Date/Time In Seconds() -> (seconds since 1Jan1904=w436:timestamp)
        n152 = local read "User ID"() -> (w437:string)
        n153 = local read "Cal Log"() -> (w427:path)
        n154 = Get Date/Time String(seconds (now)=w436) -> (date string=w434:string)  [unwired: 2 in, 1 out]
        n155 = Strip Path(path=w427) -> (stripped path=w429:path)  [unwired: 1 out]
        n156 = property on="Start Trauma" class="Bool"("Visible"=FALSE) -> ()  [unwired: 2 in, 2 out]
        n157 = call "FileIO-File or Folder Exists.vi"("path"=w429) -> ("Directory?"=w428:bool, "dup path"=w426:path)  [unwired: 7 in, 2 out]
        n158 = Format Into String(format string="%s\t%s\t%.2f\n", w437, w434, w435) -> (resulting string=w438:string)  [unwired: 2 in, 1 out]
        n159 = case shown="False" w428 {
          tunnel: w426 -> [w446 _]
          tunnel: [w445 _] -> w425
          frame False {
            n160 = Create Folder(path (use dialog)=w446) -> (error out=w445:errorcluster)  [unwired: 2 in, 2 out]
          }
          frame True {
          }
        }
        n161 = Unbundle By Name(w422) -> ("Duration (min)"=w431:dbl)
        n162 = call "Append to Text File.vi"("file path"=w427, "text"=w438, "error in (no error)"=w425) -> ("error out"=w432:errorcluster)  [unwired: 11 in, 1 out]
        n163 = property on="SPL History" class="XYGraph (strict)"(error in=w432, "XScale.Maximum"=w431) -> (error out=w433:errorcluster)  [unwired: 1 in, 1 out]
        n164 = Unbundle By Name(w422) -> ("Allow Slack"=w420:bool)
        n165 = property on="ma" class="DigNum (strict)"("Visible"=FALSE) -> ()  [unwired: 2 in, 2 out]
        n166 = while {
          tunnel: w441 -> [w451]
          tunnel: [w447] -> w442
          tunnel: w433 -> [_]
          stop <- w449 stop-if-true
          n167 = Wait (ms)(milliseconds to wait=u32 250) -> ()  [unwired: 1 out]
          n168 = Get Notifier Status(notifier=w451) -> (notifier out=w447:refnum<notifier>, # waiting=w450:i32)  [unwired: 1 in, 3 out]
          n169 = Greater Than 0?(x=w450) -> (x > 0?=w449:bool)
        }
        n170 = call "TB-Init Slack.vi"("Allow Slack"=w420, "CtlRef"=w419) -> ("Slack"=w421:T3)  [unwired: 13 in]
        n171 = property on="Stop Trauma" class="Bool"("Visible"=TRUE) -> ()  [unwired: 2 in, 2 out]
        n172 = Bundle("notification"=TRUE, "Parameters out"=w422, "Slack"=w421) -> (w423:T15)  [unwired: 1 in]
        n173 = property on="Fine Control" class="Slide (strict)"("Visible"=FALSE) -> ()  [unwired: 2 in, 2 out]
        n174 = Send Notification(notification=w423, notifier=w442) -> ()  [unwired: 1 in, 2 out]
      }
      event "Stop Trauma": Value Change {
        n175 = event-data() -> ()  [unwired: 1 in, 1 out]
        n176 = call "DAQ-Abort FGV.vi"("Action"=enum16{"Default", "Init", "Abort", "1st error"}."Abort") -> ()  [unwired: 12 in, 3 out]
      }
      event "Finished": Value Change {
        n177 = event-data() -> ()  [unwired: 1 in, 1 out]
        n178 = local write "Wizard"(TB-State_Enum."Main" ("State")) -> ()
      }
      event "EXIT": Value Change {
        n179 = event-data() -> ()  [unwired: 1 in, 1 out]
      }
      event "Crown": Value Change {
        n180 = event-data() -> ("NewVal"=w464:errorcluster, "NewVal.status"=w463:bool)  [unwired: 1 in]
        n181 = property on="Start Crown" class="Bool"("Visible"=w463) -> ()  [unwired: 2 in, 2 out]
        n182 = call "Error Handler.vi"("error in (no error)"=w464) -> ()  [unwired: 13 in, 2 out]
      }
      event "Exposure": Value Change {
        n183 = event-data() -> ("NewVal"=w467:errorcluster)  [unwired: 1 in]
        n184 = call "Error Handler.vi"("error in (no error)"=w467) -> ()  [unwired: 13 in, 2 out]
        n185 = property on="Stop Trauma" class="Bool"("Visible"=FALSE) -> ()  [unwired: 2 in, 2 out]
      }
    }
    n186 = while {
      shift-right: [w222] -> _
      shift-left: w210 -> [w225]
      tunnel: w209 -> [w220]
      tunnel: w208 -> [w219]
      shift-right: [w217] -> w206
      shift-left: w207 -> [w218]
      tunnel: [w216] -> w205
      stop <- w221 stop-if-true
      n187 = Delete From Array(array=w225) -> (deleted portion=w223:string, array with subset deleted=w224:string[])  [unwired: 2 in]
      n188 = case shown="\"restore\"" w223 {
        tunnel: w224 -> [w227 w232 w243 w246 w249 w254 w259 w270 w283]
        tunnel: [w227 w232 w236 w246 w249 w251 w257 w270 w283] -> w222
        tunnel: w220 -> [_ w231 _ _ _ _ _ _ _]
        tunnel: w219 -> [_ w230 _ _ _ _ _ _ _]
        tunnel: w218 -> [w226 w229 w242 w245 w248 _ w258 w263 w274]
        tunnel: [w226 w229 w242 w245 w248 w252 w258 w263 w274] -> w217
        tunnel: [_ TRUE _ _ _ _ _ _ _] -> w216
        frame "", Default {
        }
        frame "exit" {
          n189 = Release Notifier(notifier=w230) -> ()  [unwired: 2 in, 3 out]
          n190 = Release Notifier(notifier=w231) -> ()  [unwired: 2 in, 3 out]
          n191 = call "Abort notifier.vi"() -> ()  [unwired: 6 in, 2 out]
        }
        frame "layout" {
          w241 = waveform(dbl) {"t0"=timestamp(0 s since 1904-01-01), "dt"=1.0, "Y"=[]} ("Spectrum")
          n192 = local write "Spectrum"(w241) -> ()
          n193 = local write "Waveform"(w241) -> ()
          n194 = property on="Fine Control" class="Slide (strict)"("Visible"=FALSE) -> ()  [unwired: 2 in, 2 out]
          n195 = property on="Starts" class="DigNum (strict)"("Visible"=FALSE) -> ()  [unwired: 2 in, 2 out]
          n196 = local write "Elapsed time"("") -> ()
          n197 = local write "Wizard"(TB-State_Enum."Main" ("State")) -> ()
          n198 = local write "Display"(0) -> ()
          n199 = local write "SPL History"(cluster{dbl[], dbl[]}[] [] ("SPL History")) -> ()
          n200 = Build Array (concatenate)(w243, "params visible") -> (w236:string[])
        }
        frame "params visible" {
          w244 = TRUE
          n201 = property on="Tab Control" class="TabCtl (strict)"("Visible"=w244) -> ()  [unwired: 2 in, 2 out]
          n202 = property on="Duration (min)" class="DigNum (strict)"("Visible"=w244) -> ()  [unwired: 2 in, 2 out]
          n203 = property on="dB SPL" class="DigNum (strict)"("Visible"=w244) -> ()  [unwired: 2 in, 2 out]
          n204 = property on="Waveform" class="Ring (strict)"("Visible"=w244) -> ()  [unwired: 2 in, 2 out]
        }
        frame "params hidden" {
          w247 = FALSE
          n205 = property on="Tab Control" class="TabCtl (strict)"("Visible"=w247) -> ()  [unwired: 2 in, 2 out]
          n206 = property on="Duration (min)" class="DigNum (strict)"("Visible"=w247) -> ()  [unwired: 2 in, 2 out]
          n207 = property on="dB SPL" class="DigNum (strict)"("Visible"=w247) -> ()  [unwired: 2 in, 2 out]
          n208 = property on="Waveform" class="Ring (strict)"("Visible"=w247) -> ()  [unwired: 2 in, 2 out]
        }
        frame "restore" {
          n209 = call "TB-Restore Defaults.vi"() -> ("Exposure parameters out"=w252:T4, "error out"=w253:errorcluster)  [unwired: 14 in]
          n210 = call "Error Handler.vi"("error in (no error)"=w253) -> ()  [unwired: 13 in, 2 out]
          n211 = Build Array (concatenate)(w254, string[] ["show"]) -> (w251:string[])
        }
        frame "show" {
          n212 = Build Array (concatenate)(w259, "show1", "show2") -> (w257:string[])
        }
        frame "show1" {
          n213 = Unbundle By Name(w263) -> ("Low cutoff (kHz)"=w264:dbl, "High cutoff (kHz)"=w265:dbl, "Freq (kHz)"=w260:dbl, "Duration (min)"=w266:dbl, "dB SPL"=w267:dbl, "refWav"=w269:path, "WAVfile"=w268:path, "Waveform"=w262:enum16{"Noise", "File", "Tone"})
          n214 = case shown="\"File\"" w262 {
            tunnel: [enum32{"Tone", "Noise", "File"}."Noise" ("Tab Control") enum32{"Tone", "Noise", "File"}."File" ("Tab Control") enum32{"Tone", "Noise", "File"}."Tone" ("Tab Control")] -> w261
            frame "Noise", Default {
            }
            frame "File" {
            }
            frame "Tone" {
            }
          }
          n215 = local write "Low cutoff (kHz)"(w264) -> ()
          n216 = local write "High cutoff (kHz)"(w265) -> ()
          n217 = local write "Frequency (kHz)"(w260) -> ()
          n218 = local write "Duration (min)"(w266) -> ()
          n219 = local write "dB SPL"(w267) -> ()
          n220 = local write "WAVfile"(w268) -> ()
          n221 = local write "refWAV"(w269) -> ()
          n222 = local write "Waveform"(w262) -> ()
          n223 = local write "Tab Control"(w261) -> ()
        }
        frame "show2" {
          n224 = Unbundle By Name(w274) -> ("Fine adjust.Max"=w278:dbl, "Fine adjust.Min"=w279:dbl, "Mic gain"=w282:dbl)
          n225 = Unbundle By Name(w274) -> ("use mic correction"=w276:bool, "micCorrFile"=w275:path)
          n226 = Add(x=w278, y=w279) -> (x+y=w277:dbl)
          n227 = local write "B&K Mic Gain"(w282) -> ()
          n228 = local write "Use mic correction"(w276) -> ()
          n229 = property on="micCorrFile" class="Path"("Value"=w275, "Visible"=w276) -> ()  [unwired: 2 in, 2 out]
          n230 = Divide(x=w277, y=2.0) -> (x/y=w280:dbl)
          n231 = property on="Fine Control" class="Slide (strict)"("Scale.Maximum"=w278, "Scale.Minimum"=w279, "Value"=w280) -> ()  [unwired: 2 in, 2 out]
        }
      }
      n232 = Empty Array?(array=w222) -> (empty?=w221:bool)
    }
  }
  n233 = while {
    tunnel: w7 -> [w473]
    stop <- w472 stop-if-true
    # "PISTONPHONE MEASUREMENT"
    n234 = Wait on Notification(notifier=w473, ignore previous (F)=TRUE) -> (notification=w471:T4, error out=w472:errorcluster)  [unwired: 2 in, 2 out]
    n235 = case shown="No Error" w472 {
      tunnel: w471 -> [w484 _]
      frame No Error {
        n236 = call "TB-Initialize Pistonphone Measurement.vi"("Exposure parameters"=w484) -> ("Params thru"=w483:T4, "error out"=w480:errorcluster)  [unwired: 13 in]
        n237 = call "AIDI-Engine.vi"("Action"=AIDI-Action."Init & Start", "error in (no error)"=w480) -> ("error out"=w479:errorcluster)  [unwired: 10 in, 3 out]
        n238 = call "AIDI-Engine.vi"("Action"=AIDI-Action."Read", "error in (no error)"=w479) -> ("AI"=w478:dbl[][], "error out"=w476:errorcluster)  [unwired: 10 in, 2 out]
        n239 = call "AIDI-Engine.vi"("Action"=AIDI-Action."Clean up", "error in (no error)"=w476) -> ("error out"=w475:errorcluster)  [unwired: 10 in, 3 out]
        n240 = case shown="No Error" w475 {
          selector: w475 -> [_ w503]
          tunnel: w478 -> [w502 _]
          tunnel: [w489 w503] -> w486
          tunnel: w483 -> [w488 _]
          frame No Error {
            n241 = Index Array(array=w502) -> (element=w498:dbl[])  [unwired: 2 in]
            "Pistonphone\nWaveform" <- w498
            n242 = call-poly <vilib>:"Mean.vi"("X"=w498) -> ("mean"=w497:dbl)  [unwired: 1 out]
            n243 = call "Range.vi"("Array"=w498) -> ("Range"=w501:dbl)
            n244 = Greater?(x=w501, y=6.0) -> (0:→"Overload":bool)
            n245 = Subtract(x=w498, y=w497) -> (x-y=w490:dbl[])
            n246 = Unbundle By Name(w488) -> ("Mic gain"=w487:dbl)
            n247 = call-poly <vilib>:"RMS.vi"("X"=w490) -> ("rms value"=w496:dbl)  [unwired: 1 out]
            n248 = local read "User ID"() -> (w491:string)
            n249 = Divide(x=w496, y=1e-06) -> (x/y=w494:dbl)
            n250 = call-poly "Linear to dB.vi"("Linear"=w494) -> ("dB"=w493:dbl)
            n251 = call "TB-Save Cal Signal.vi"("Params"=w488, "ID"=w491, "Mic signal"=w490) -> ("error out"=w489:errorcluster)  [unwired: 12 in]
            n252 = Subtract(x=w493, y=w487) -> (x-y=→"Calibrator Voltage\n(dB rms re 1 uV)" →"Pistonphone Factor":dbl)
          }
          frame Error {
          }
        }
        n253 = call "Error Handler.vi"("error in (no error)"=w486) -> ("error?"=w485:bool)  [unwired: 13 in, 1 out]
        n254 = flat-sequence {
          tunnel: w485 -> [_]
          frame #0 {
            n255 = property on="Next" class="Bool"("Visible"=TRUE) -> ()  [unwired: 2 in, 2 out]
          }
        }
      }
      frame Error {
      }
    }
  }
  n256 = disable-structure shown="RUN_TIME_ENGINE==True" {
    disable-tunnel: w6 -> [w505 _]
    frame condition #0 {
      n257 = Quit LabVIEW(quit? (T)=w505) -> ()
    }
    frame condition #1 (active) {
    }
  }
